vi "ma_HasIIRSpecsChanged.vi"(4 "optional IIR filter specifications":T1={"Lower PB"=100.0, "Upper PB"=0.0, "Lower SB"=200.0, "Upper SB"=0.0, "PB Gain"=-3.0, "SB Gain"=-60.0, "Scale"=TRUE} {"PB Gain" format="%0.2f"; "SB Gain" format="%0.2f"; "Lower SB" format="%0.2p"; "Upper SB" format="%0.2f"; "Lower PB" format="%0.2p"; "Upper PB" format="%0.2f"}, 6 "IIR filter specifications":T2={"Topology"=enum."Off", "Type"=enum."Lowpass", "Order"=1, "Lower Fc"=100.0, "Upper Fc"=200.0, "PB Ripple"=1.0, "SB Attenuation"=60.0} {"PB Ripple" format="%0.2f"; "Lower Fc" format="%0.2p"; "SB Attenuation" format="%0.2f"; "Upper Fc" format="%0.2p"}, 8 "error in (no error)":errorcluster, 10 "redesign filter":bool) -> (0 "error out":errorcluster, 3 "ValsDifferent?":bool)   [LabVIEW 2020, in "NI_MAPro.lvlib"]
uses:
  NI_MAPro.lvlib
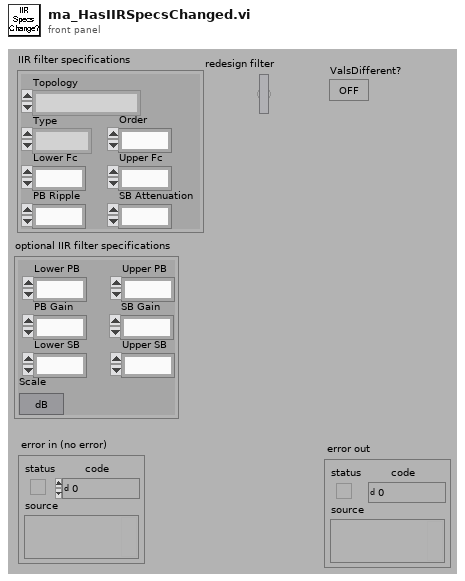
[diagram p1: front panel]
types:
  T1 = cluster{"Lower PB":dbl, "Upper PB":dbl, "Lower SB":dbl, "Upper SB":dbl, "PB Gain":dbl, "SB Gain":dbl, "Scale":bool}
  T2 = cluster{"Topology":enum16{"Off", "Butterworth", "Chebyshev", "Inverse Chebyshev", "Elliptic", "Bessel"}, "Type":enum16{"Lowpass", "Highpass", "Bandpass", "Bandstop"}, "Order":i32, "Lower Fc":dbl, "Upper Fc":dbl, "PB Ripple":dbl, "SB Attenuation":dbl}
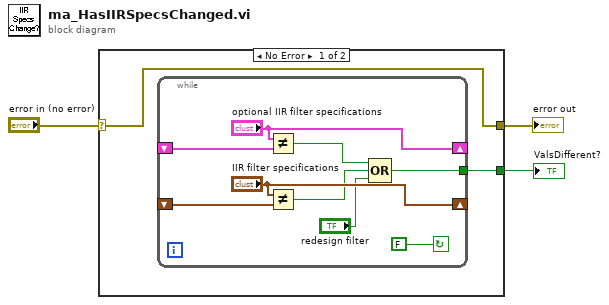
[diagram p0: block diagram]
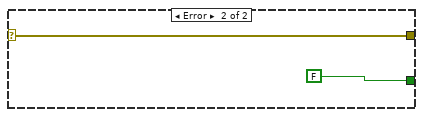
[diagram p2: hidden frame]
diagram:
  n1 = case shown="No Error" "error in (no error)" {
    selector: "error in (no error)" -> [w4 w15]
    tunnel: [w5 FALSE] -> w2
    tunnel: [w4 w15] -> w1
    frame No Error {
      n2 = while {
        shift-left: _ -> [w13]
        shift-right: ["IIR filter specifications"] -> _
        tunnel: [w7] -> w5
        shift-left: _ -> [w11]
        shift-right: ["optional IIR filter specifications"] -> _
        stop <- FALSE continue-if-true
        n3 = Not Equal?(x="optional IIR filter specifications", y=w11) -> (x != y?=w9:bool)
        n4 = Not Equal?(x="IIR filter specifications", y=w13) -> (x != y?=w8:bool)
        n5 = Compound Arithmetic op=OR(w9, w8, "redesign filter") -> (w7:bool)
      }
    }
    frame Error {
    }
  }
  "error out" <- w1
  "ValsDifferent?" <- w2
